vi "test_send.vi"() -> ()   [LabVIEW 2018]
uses:
  <vilib>/myRIO/Instrument Drivers/Onboard IO/AO/typedefs/AO Reference.ctl
  <vilib>/myRIO/Common/Instrument Driver Framework/Utilities/typedefs/myRIO Generic Hardware Reference.ctl
  <vilib>/myRIO/Common/Instrument Driver Framework/Utilities/typedefs/Hardware Version Enum.ctl
  <vilib>/myRIO/Common/Instrument Driver Framework/Utilities/typedefs/myRIO v1.0 Reference.ctl
  <vilib>/myRIO/Common/Instrument Driver Framework/Utilities/typedefs/Generic FPGA Reference.ctl
  <vilib>/myRIO/Common/Instrument Driver Framework/myRIO v1.0/AO/typedefs/AO Channels List.ctl
  <vilib>/myRIO/Common/Instrument Driver Framework/myRIO v1.0/AO/typedefs/AO Channels Enum.ctl
  <vilib>/myRIO/Common/Instrument Driver Framework/Utilities/typedefs/Analog Scaling Constants List.ctl
  <vilib>/myRIO/Common/Instrument Driver Framework/Utilities/typedefs/Analog Scaling Constants.ctl
  <vilib>/userdefined/High Color/nirio_resource_hc.ctl
  <vilib>/myRIO/Common/Instrument Driver Framework/ELVIS III v1.0/AO/vis/ELVIS III v1.1 Open AO.vi
  <vilib>/myRIO/Common/Instrument Driver Framework/Utilities/vis/Validate Channels.vi
  <vilib>/myRIO/Common/Instrument Driver Framework/ELVIS III v1.0/AO/vis/ELVIS III v1.0 Reserve AO.vi
  <vilib>/myRIO/Common/Instrument Driver Framework/ELVIS III v1.0/AO/vis/ELVIS III v1.0 Close AO.vi
  <vilib>/myRIO/Common/Instrument Driver Framework/ELVIS III v1.0/AO/vis/ELVIS III v1.0 Build MUX Configuration AO.vi
  <vilib>/myRIO/Common/Instrument Driver Framework/ELVIS III v1.0/Resource Manager/vis/ELVIS III v1.0 Reserve Channel List.vi
  <vilib>/myRIO/Common/Instrument Driver Framework/ELVIS III v1.0/AO/vis/ELVIS III v1.0 Unreserve AO.vi
  <vilib>/myRIO/Common/Instrument Driver Framework/ELVIS III v1.0/Resource Manager/vis/ELVIS III v1.0 Reserve Channel.vi
  <vilib>/myRIO/Common/Instrument Driver Framework/ELVIS III v1.0/Resource Manager/vis/ELVIS III v1.0 Unreserve Channel.vi
  <vilib>/myRIO/Common/Instrument Driver Framework/ELVIS III v1.0/Resource Manager/vis/ELVIS III v1.0 Unreserve Channel List.vi
  <vilib>/myRIO/Common/Instrument Driver Framework/ELVIS III v1.0/Resource Manager/vis/ELVIS III v1.0 Build Mutex Name.vi
  <vilib>/Utility/VariantDataType/GetNumericInfo.vi
  <vilib>/Utility/error.llb/Error Cluster From Error Code.vi
  <vilib>/myRIO/Common/Instrument Driver Framework/ELVIS III v1.0/ELVIS III v1.1 Open.vi
  <vilib>/myRIO/Common/Instrument Driver Framework/Utilities/vis/IO Manager.vi
  <vilib>/myRIO/Common/Instrument Driver Framework/Utilities/vis/Configuration Manager.vi
  <vilib>/myRIO/Common/Instrument Driver Framework/myRIO v1.0/myRIO v1.0 Close.vi
  <vilib>/myRIO/Common/Instrument Driver Framework/ELVIS III v1.0/AO/vis/ELVIS III v1.0 Write AO.vi
  <vilib>/myRIO/Instrument Drivers/Onboard IO/AO/vis/myRIO AO Open.xnode
  <vilib>/myRIO/Instrument Drivers/Onboard IO/AO/AO.lvlib
panel:
  in  "Stop":bool
  in  "Input String":string
  in  "Send Message":bool
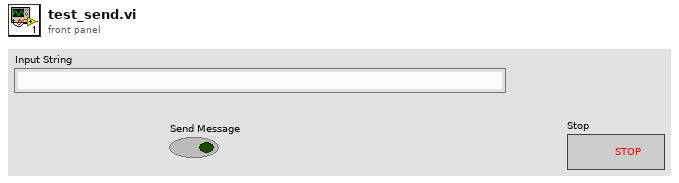
[diagram p1: front panel]
types:
  T1 = typedef "AO.lvlib/AO Reference.ctl" = cluster{"myRIO Reference":T2, "AO Channel List":T6, "AO Scaling Constant List":T8}
  T2 = typedef "myRIO Generic Hardware Reference.ctl" = cluster{"myRIO Model":T3, "myRIO Hardware Reference":T4}
  T3 = typedef "Hardware Version Enum.ctl" = enum16{"Unknown", "myRIO-1900", "myRIO-1950", "roboRIO", "NI ELVIS RIO CM", "ELVIS III"}
  T4 = typedef "myRIO v1.0 Reference.ctl" = cluster{"Generic FPGA Reference":T5, "Allow multiple opens":bool}
  T5 = typedef "Generic FPGA Reference.ctl" = refnum<k20>
  T6 = typedef "AO Channels List.ctl" = T7[]
  T7 = typedef "AO Channels Enum.ctl" = enum16{"Not Connected", "AudioOut/Left", "AudioOut/Right", "C/AO0", "C/AO1", "A/AO0", "A/AO1", "B/AO0", "B/AO1"}
  T8 = typedef "Analog Scaling Constants List.ctl" = T9[]
  T9 = typedef "Analog Scaling Constants.ctl" = cluster{"LSB Weight (Volts)":dbl, "Offset (Volts)":dbl, "Signed?":bool}
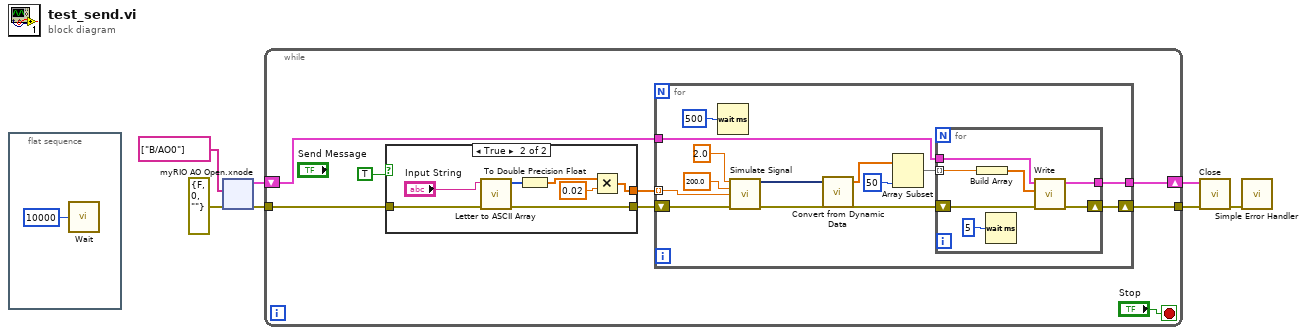
[diagram p0: block diagram]
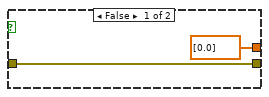
[diagram p2: hidden frame]
diagram:
  n1 = flat-sequence {
    frame #0 {
      n2 = call "Wait"("Count(mSec)"=u32 10000) -> ()  [unwired: 1 out]
    }
  }
  n3 = xnode "myRIO AO Open.xnode"("error in (no error)"=errorcluster {"status"=FALSE, "code"=0, "source"=""}, "Channel Names"=tag[] ["B/AO0"]) -> ("error out"=w7:errorcluster, "AO Ref Out"=w6:T1)  [unwired: 1 in]
  n4 = while {
    tunnel: [w15] -> w2
    shift-right: [w11] -> w3
    shift-left: w6 -> [w16]
    tunnel: w7 -> [w10]
    stop <- "Stop" stop-if-true
    n5 = case shown="True" TRUE {
      tunnel: [w17 w20] -> w13
      tunnel: [dbl[] [0.0] w19] -> w12
      tunnel: w10 -> [w17 w21]
      frame False {
      }
      frame True {
        n6 = call "Letter to ASCII Array.vi"("error in (no error)"=w21, "Input String"="Input String") -> ("error out"=w20:errorcluster, "String to ASCII Array"=w22:u8[])  [unwired: 8 in]
        n7 = To Double Precision Float(number=w22) -> (double precision float=w25:dbl[])
        n8 = Multiply(x=w25, y=0.02) -> (x*y=w19:dbl[])
      }
    }
    n9 = for {
      tunnel: w16 -> [w38]
      shift-right: [w36] -> w15
      shift-left: w13 -> [w31]
      tunnel: w12 -> [w28] mode=indexing
      tunnel: [w26] -> w11
      n10 = Wait (ms)(milliseconds to wait=u32 500) -> ()  [unwired: 1 out]
      n11 = call "Simulate Signal"("Offset"=2.0, "Frequency"=200.0, "Amplitude"=w28, "error in (no error)"=w31) -> ("Sine"=w37:dynamicdata, "error out"=w30:errorcluster)  [unwired: 10 in]
      n12 = call "Convert from Dynamic Data"("Dynamic Data Type"=w37) -> ("Array"=w34:dbl[])  [unwired: 3 in]
      n13 = Array Subset(array=w34, length=50) -> (w32:dbl[])  [unwired: 1 in]
      n14 = for {
        tunnel: w38 -> [w45]
        shift-right: [w41] -> w36
        shift-left: w30 -> [w44]
        tunnel: w32 -> [w43] mode=indexing
        tunnel: [w39] -> w26
        n15 = Build Array(w43) -> (w42:dbl[])
        n16 = Wait (ms)(milliseconds to wait=u32 5) -> ()  [unwired: 1 out]
        n17 = call <vilib>:"Write.vi"("error in (no error)"=w44, "Values"=w42, "AO Ref In"=w45) -> ("error out"=w41:errorcluster, "AO Ref Out"=w39:T1)  [unwired: 6 in]
      }
    }
  }
  n18 = call <vilib>:"Close.vi"("error in (no error)"=w2, "AO Ref In"=w3) -> ("error out"=w1:errorcluster)  [unwired: 9 in]
  n19 = call <vilib>:"Simple Error Handler.vi"("error in (no error)"=w1) -> ()  [unwired: 4 in, 5 out]
